vi "Actuators Get Position Channel.vi"(0 "Notifier Name":string, 7 "Channel":i32, 11 "Error In":errorcluster) -> (4 "Notifier Name Out":string, 6 "Position":dbl, 8 "Status Bits":u32, 10 "Moving":bool, 15 "Error Out":errorcluster)   [LabVIEW 2020]
uses:
  Actuators Controls/Actuators Note Type.ctl
  Actuators Controls/Actuators Actions.ctl
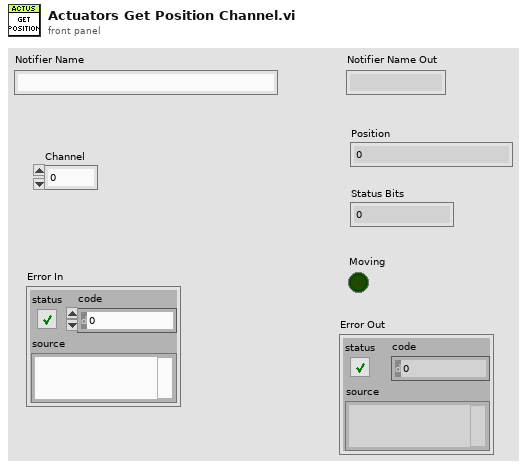
[diagram p1: front panel]
types:
  T1 = typedef "Actuators Note Type.ctl" = cluster{"Actions":T2, "Cmd Received ":bool, "Setpoint":dbl[], "Position":dbl[], "Channel":i32[], "Jog Step":dbl[], "Velocity":dbl[], "Acceleration":dbl[], "Status Bits":u32[], "Moving":bool[]}
  T2 = typedef "Actuators Actions.ctl" = enum16{"Nothing", "Get Position", "Get Acceleration", "Get Velocity", "Get Jog Step", "Set Acceleration", "Set Velocity", "Set Jog Step", "Move Absolute", "Move Relative", "Jog Forward", "Jog Reverse", "Set Moving", "Halt", "Quit"}
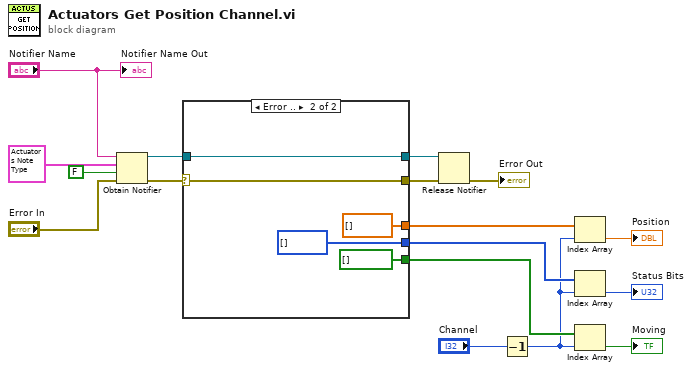
[diagram p0: block diagram]
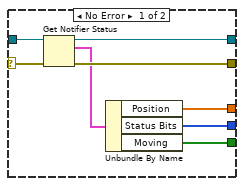
[diagram p2: hidden frame]
diagram:
  n1 = Obtain Notifier(name (unnamed)="Notifier Name", notification data type=T1 {"Actions"=enum."Nothing", "Cmd Received "=FALSE, "Setpoint"=[], "Position"=[], "Channel"=[], "Jog Step"=[], "Velocity"=[], "Acceleration"=[], "Status Bits"=[], "Moving"=[]} ("Actuators Note"), create if not found? (T)=FALSE, error in (no error)="Error In") -> (notifier out=w13:refnum<notifier>, error out=w16:errorcluster)  [unwired: 1 out]
  n2 = case shown="Error .." w16 {
    selector: w16 -> [w24 w29]
    tunnel: w13 -> [w25 w30]
    tunnel: [w23 w30] -> w12
    tunnel: [w22 w29] -> w11
    tunnel: [w20 dbl[] [] ("Position")] -> w8
    tunnel: [w19 u32[] [] ("Status Bits")] -> w7
    tunnel: [w18 bool[] [] ("Moving")] -> w6
    frame No Error {
      n3 = Get Notifier Status(notifier=w25, error in (no error)=w24) -> (notifier out=w23:refnum<notifier>, current notification=w21:T1, error out=w22:errorcluster)  [unwired: 2 out]
      n4 = Unbundle By Name(w21) -> ("Position"=w20:dbl[], "Status Bits"=w19:u32[], "Moving"=w18:bool[])
    }
    frame Error {
    }
  }
  n5 = Release Notifier(notifier=w12, error in (no error)=w11) -> (error out=→"Error Out":errorcluster)  [unwired: 1 in, 2 out]
  n6 = Decrement(x="Channel") -> (x-1=w4:i32)
  n7 = Index Array(array=w8, index=w4) -> (element=→"Position":dbl)
  n8 = Index Array(array=w7, index=w4) -> (element=→"Status Bits":u32)
  n9 = Index Array(array=w6, index=w4) -> (element=→"Moving":bool)
  "Notifier Name Out" <- "Notifier Name"
